vi "Pow Meas Configure and Measure.vi"(0 "task/channels in":refnum<k21>, 5 "Channel Settings":T2={"Current Setpoint"=3.0, "Voltage Setpoint"=6.0}, 7 "Timing Settings":T4={"Sample Clock Source"="OnboardClock", "Sample Rate"=1000.0, "Number of Samples"=100} {"Number of Samples" format="%0.2f"}, 9 "Trigger Settings":T3={"Digital Start Trigger?"=FALSE, "Digital Start Trigger Source"="/TS1Mod2/PFI0", "Digital Start Trigger Edge"=10280} {"Digital Start Trigger Edge" items=["Rising"=10280, "Falling"=10171]}, 11 "error in (no error)":errorcluster, 13 "Operation":T5, 14 "Calculate Analysis?":bool) -> (4 "task out":refnum<k21>, 6 "voltage":dbl[](array[numeric]) format="%.2f", 8 "Current":dbl[](array[numeric]) format="%.2f", 10 "Analyzed Data":T1, 15 "error out":errorcluster)   [LabVIEW 2021, in "Power Measurement.lvlib"]
uses:
  Power Measurement.lvlib
  Typedefs/pow Meas Configure or Measure.ctl
  Typedefs/Pow Meas Timing Settings.ctl
  Typedefs/Pow Meas Rigger Settings.ctl
  Typedefs/Pow Meas Init Settings.ctl
  Typedefs/Pow Meas Analyzed Data.ctl
  <vilib>/DAQmx/read.llb/DAQmx Read (Power 1D DBL 1Chan NSamp).vi
  <vilib>/DAQmx/configure/timing.llb/DAQmx Timing (Sample Clock).vi
  <vilib>/DAQmx/configure/trigger.llb/DAQmx Start Trigger (Digital Edge).vi
  <vilib>/DAQmx/miscellaneous.llb/DAQmx Fill In Error Info.vi
  <resource>/objmgr/daqmx.rc
  Main Library.lvlib
panel:
  out "Actual Sample Rate":dbl=1000.0 format="%0.2f"
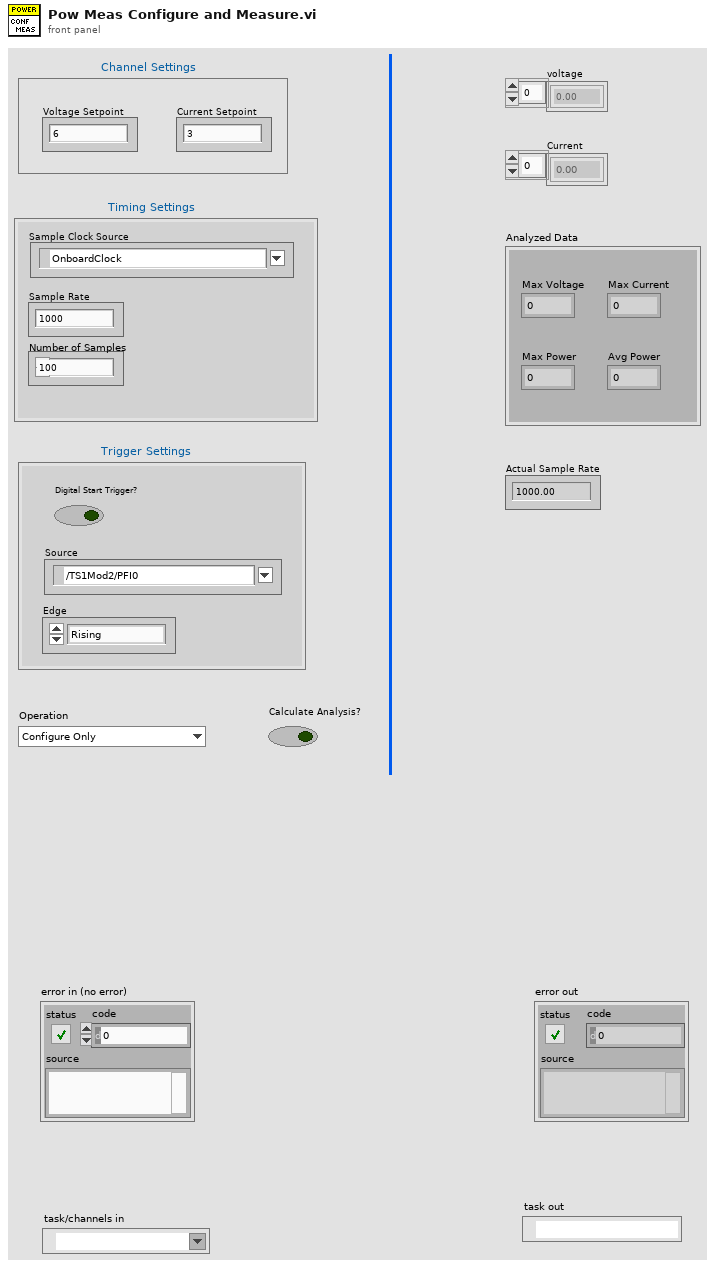
[diagram p1: front panel]
types:
  T1 = typedef "Main Library.lvlib/Pow Meas Analyzed Data.ctl" = cluster{"Max Voltage":dbl, "Max Current":dbl, "Max Power":dbl, "Avg Power":dbl}
  T2 = typedef "Power Measurement.lvlib/Pow Meas Init Settings.ctl" = cluster{"Current Setpoint":dbl, "Voltage Setpoint":dbl}
  T3 = typedef "Power Measurement.lvlib/Pow Meas Rigger Settings.ctl" = cluster{"Digital Start Trigger?":bool, "Digital Start Trigger Source":tag, "Digital Start Trigger Edge":i32}
  T4 = typedef "Power Measurement.lvlib/Pow Meas Timing Settings.ctl" = cluster{"Sample Clock Source":tag, "Sample Rate":dbl, "Number of Samples":i32}
  T5 = typedef "Power Measurement.lvlib/pow Meas Configure or Measure.ctl" = enum16{"Configure Only", "Measure Only", "Configure and Measure"}
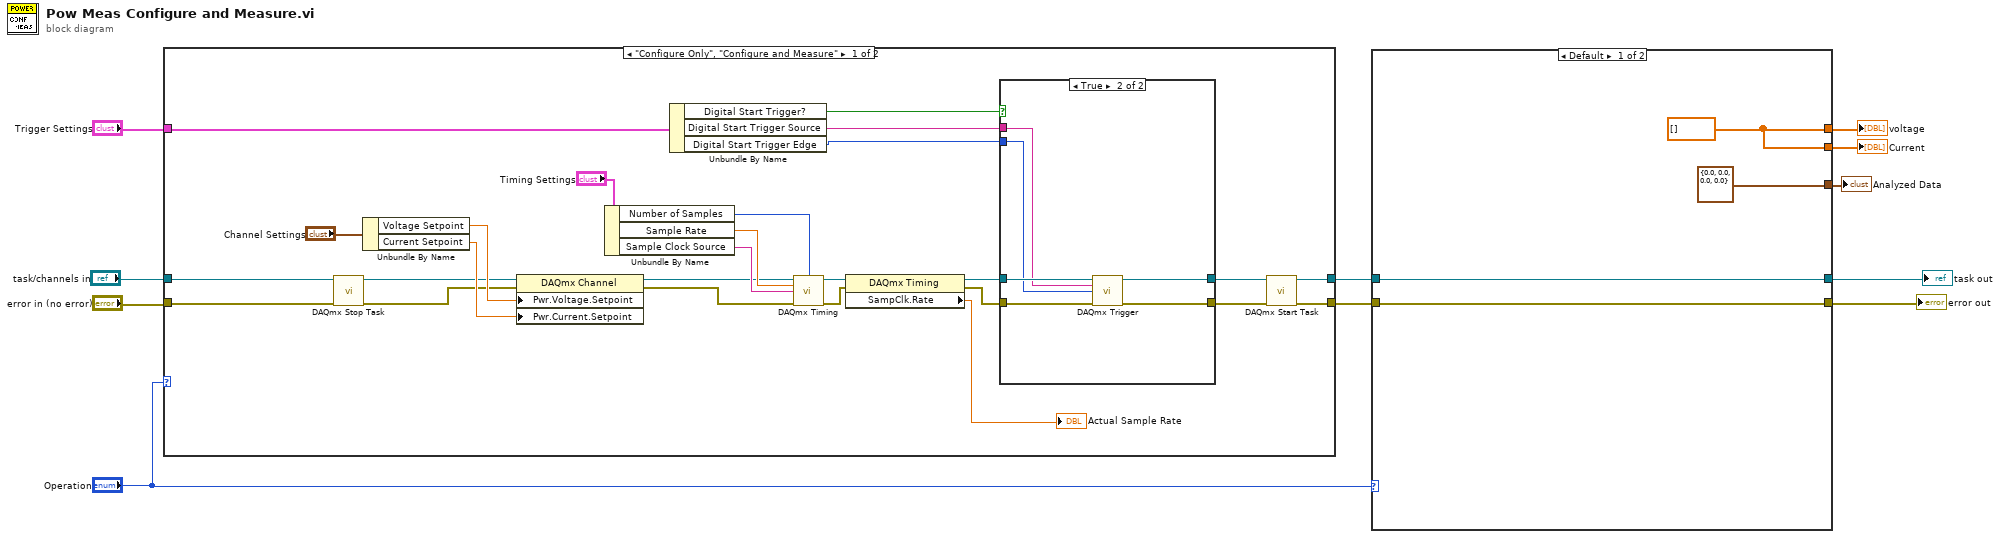
[diagram p0: block diagram]
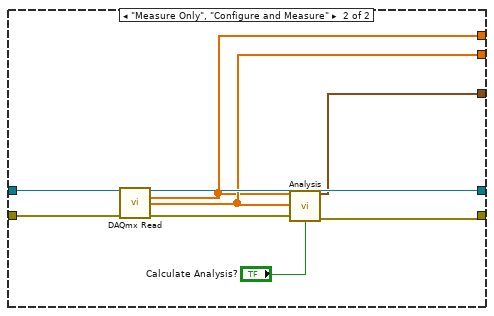
[diagram p2: hidden frame]
diagram:
  n1 = case shown="\"Configure Only\", \"Configure and Measure\"" "Operation" {
    tunnel: "task/channels in" -> [w15 w47]
    tunnel: "error in (no error)" -> [w12 w46]
    tunnel: "Trigger Settings" -> [w29 _]
    tunnel: [w23 w46] -> w7
    tunnel: [w22 w47] -> w6
    frame "Configure Only", "Configure and Measure" {
      n2 = call <vilib>:"DAQmx Stop Task.vi"("task/channels in"=w15, "error in"=w12) -> ("task out"=w14:refnum<k21>, "error out"=w13:errorcluster)  [unwired: 12 in]
      n3 = Unbundle By Name("Channel Settings") -> ("Voltage Setpoint"=w18:dbl, "Current Setpoint"=w16:dbl)
      n4 = property class="DAQmx Channel"(reference=w14, error in=w13, "Pwr.Voltage.Setpoint"=w18, "Pwr.Current.Setpoint"=w16) -> (reference out=w17:refnum<k21>, error out=w19:errorcluster)
      n5 = Unbundle By Name("Timing Settings") -> ("Number of Samples"=w35:i32, "Sample Rate"=w37:dbl, "Sample Clock Source"=w36:tag)
      n6 = Unbundle By Name(w29) -> ("Digital Start Trigger?"=w28:bool, "Digital Start Trigger Source"=w27:tag, "Digital Start Trigger Edge"=w26:i32)
      n7 = call-poly <vilib>:"DAQmx Timing.vi"("task/channels in"=w17, "samples per channel"=w35, "rate"=w37, "source"=w36, "error in"=w19) -> ("task out"=w34:refnum<k21>, "error out"=w33:errorcluster)  [unwired: 9 in]
      n8 = property class="DAQmx Timing"(reference=w34, error in=w33) -> (reference out=w30:refnum<k21>, error out=w31:errorcluster, "SampClk.Rate"=→"Actual Sample Rate":dbl)
      n9 = case shown="True" w28 {
        tunnel: w31 -> [w39 w45]
        tunnel: w30 -> [w38 w44]
        tunnel: [w39 w43] -> w25
        tunnel: w27 -> [_ w42]
        tunnel: w26 -> [_ w41]
        tunnel: [w38 w40] -> w24
        frame False {
        }
        frame True {
          n10 = call-poly <vilib>:"DAQmx Trigger.vi"("task/channels in"=w44, "source"=w42, "edge"=w41, "error in"=w45) -> ("task out"=w40:refnum<k21>, "error out"=w43:errorcluster)  [unwired: 10 in]
        }
      }
      n11 = call <vilib>:"DAQmx Start Task.vi"("task/channels in"=w24, "error in"=w25) -> ("task out"=w22:refnum<k21>, "error out"=w23:errorcluster)  [unwired: 12 in]
    }
    frame Default {
    }
  }
  n12 = case shown="Default" "Operation" {
    tunnel: w7 -> [w50 w58]
    tunnel: w6 -> [w51 w59]
    tunnel: [w51 w60] -> w5
    tunnel: [w50 w55] -> w4
    tunnel: [T1 {"Max Voltage"=0.0, "Max Current"=0.0, "Max Power"=0.0, "Avg Power"=0.0} ("Analyzed Data") w54] -> w3
    tunnel: [w48 w53] -> w2
    tunnel: [w48 w52] -> w1
    frame Default {
      w48 = dbl[] [] ("voltage")
    }
    frame "Measure Only", "Configure and Measure" {
      n13 = call-poly <vilib>:"DAQmx Read.vi"("task/channels in"=w59, "error in"=w58) -> ("task out"=w60:refnum<k21>, "voltage"=w52:dbl[], "current"=w53:dbl[], "error out"=w56:errorcluster)  [unwired: 10 in]
      n14 = call "Analysis.vi"("Voltage"=w52, "Current"=w53, "error in (no error)"=w56, "Create Analysis?"="Calculate Analysis?") -> ("Analyzed Data"=w54:T1, "error out"=w55:errorcluster)  [unwired: 10 in]
    }
  }
  "error out" <- w4
  "task out" <- w5
  "Analyzed Data" <- w3
  "voltage" <- w1
  "Current" <- w2
